vi "SeparateString.vi"(11 "strArrayIn":string[](array[string])) -> (1 "strArrayOut":string[](array[string]), 2 "mu32ArrayOut":u32[](array[numeric]), 3 "strArrayBuf":string[](array[string]))   [LabVIEW 2011]
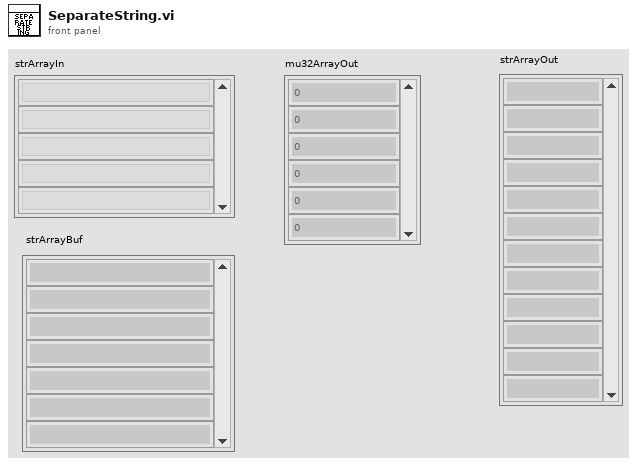
[diagram p1: front panel]
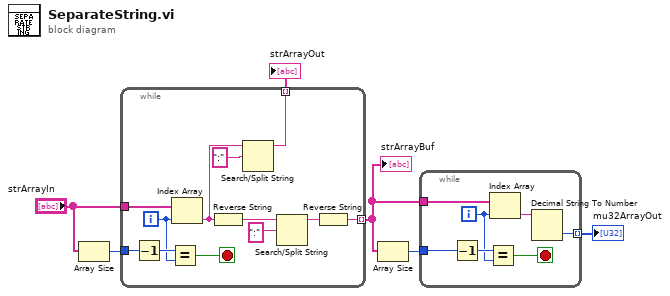
[diagram p0: block diagram]
diagram:
  n1 = Array Size(array="strArrayIn") -> (size(s)=w6:i32)
  n2 = while {
    tunnel: w6 -> [w17]
    tunnel: "strArrayIn" -> [w15]
    tunnel: [w10] -> w2 mode=indexing
    tunnel: [w7] -> w1 mode=indexing
    i -> [w11]
    stop <- w18 stop-if-true
    n3 = Decrement(x=w17) -> (x-1=w16:i32)
    n4 = Equal?(x=w16, y=w11) -> (x = y?=w18:bool)
    n5 = Index Array(array=w15, index=w11) -> (element=w9:string)
    n6 = Reverse String(1:w9) -> (0:w14:string)
    n7 = Search/Split String(string=w9, search string/char (-)=":" ("搜索字符串/字符(-)")) -> (substring before match=w7:string)  [unwired: 1 in, 2 out]
    n8 = Search/Split String(string=w14, search string/char (-)=":" ("搜索字符串/字符(-)")) -> (substring before match=w12:string)  [unwired: 1 in, 2 out]
    n9 = Reverse String(1:w12) -> (0:w10:string)
  }
  "strArrayBuf" <- w2
  "strArrayOut" <- w1
  n10 = Array Size(array=w2) -> (size(s)=w4:i32)
  n11 = while {
    tunnel: w4 -> [w25]
    tunnel: w2 -> [w21]
    tunnel: [w19] -> w3 mode=indexing
    i -> [w22]
    stop <- w23 stop-if-true
    n12 = Decrement(x=w25) -> (x-1=w24:i32)
    n13 = Equal?(x=w24, y=w22) -> (x = y?=w23:bool)
    n14 = Index Array(array=w21, index=w22) -> (element=w20:string)
    n15 = Decimal String To Number(string=w20) -> (number=w19:i32)  [unwired: 2 in, 1 out]
  }
  "mu32ArrayOut" <- w3
